vi "Handle Error.vi"(8 "error in (no error)":errorcluster, 11 "WebSocket Server in":refnum<class "WebSocket Server.lvclass">) -> (0 "error out":errorcluster, 2 "stop actor?":bool=TRUE, 3 "WebSocket Server out":refnum<class "WebSocket Server.lvclass">)   [LabVIEW 2021, in "WebSocket Actors.lvlib" / "WebSocket Server.lvclass"]
doc: "(<B>Filename</B>: Actor Framework.lvlib:Actor.lvclass:Handle Error.vi)\n\nDefines how the actor handles an error that occurred while processing a message. By default, this method does nothing except stop the actor."
uses:
  WebSocket Server.lvclass
  C:/Program Files/National Instruments/LabVIEW 2021/vi.lib/ActorFramework/Actor/Actor.lvclass
  <vilib>/ActorFramework/Actor/Actor.lvclass/Actor.ctl
  WebSocket Server.lvclass/WebSocket Server.ctl
  <vilib>/ActorFramework/Report Error Msg/Report Error Msg.lvclass/Report Error Msg.ctl
  <vilib>/ActorFramework/Message Enqueuer/Message Enqueuer.lvclass/Message Enqueuer.ctl
  Read Subscriber Enqueuer.vi
  <vilib>/ActorFramework/Message Enqueuer/Enqueue.vi
  <vilib>/ActorFramework/Message Enqueuer/Equals Not A Refnum.vi
  <vilib>/ActorFramework/Actor/Read Caller Enqueuer.vi
  <vilib>/ActorFramework/Report Error Msg/Report Error Msg.lvclass
  C:/Program Files/National Instruments/LabVIEW 2021/vi.lib/ActorFramework/Message/Message.lvclass
  <vilib>/Utility/LVClass/Get LV Class Name.vi
  <resource>/AFDebug/Generate Trace for Message.vi
  <vilib>/ActorFramework/Message Priority Queue/Priority Enqueue.vi
  <vilib>/ActorFramework/Message Enqueuer/Message Enqueuer.lvclass
  <userlib>/_OpenG.lib/error/error.llb/openg_error.lvlib
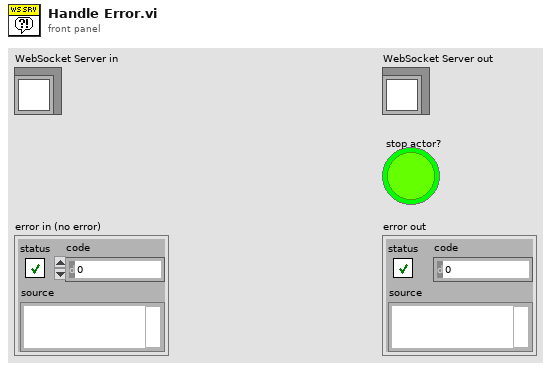
[diagram p1: front panel]
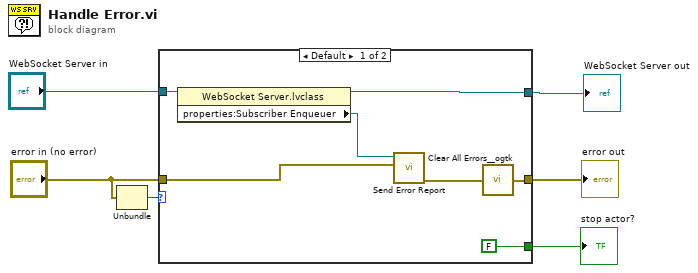
[diagram p0: block diagram]
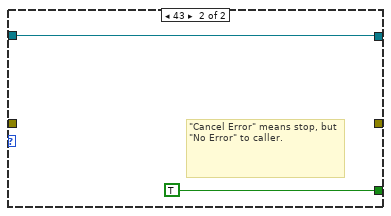
[diagram p2: hidden frame]
diagram:
  n1 = Unbundle("error in (no error)") -> ("code"=w6:i32)  [unwired: 2 out]
  n2 = case shown="Default" w6 {
    tunnel: [w8 _] -> w4
    tunnel: "error in (no error)" -> [w13 _]
    tunnel: [FALSE ("stop actor?") TRUE ("stop actor?")] -> w3
    tunnel: "WebSocket Server in" -> [w11 w14]
    tunnel: [w10 w14] -> w1
    frame Default {
      n3 = property class="WebSocket Server.lvclass"(reference=w11) -> (reference out=w10:refnum<class "WebSocket Server.lvclass">, "properties:Subscriber Enqueuer"=w9:refnum<class "Message Enqueuer.lvclass">)  [unwired: 1 in, 1 out]
      n4 = call <vilib>:"Send Error Report.vi"("Error From Sender"=w13, "Message Enqueuer"=w9) -> ("error out"=w7:errorcluster)  [unwired: 9 in]
      n5 = call <userlib>:"Clear All Errors__ogtk.vi"("Error In"=w7) -> ("Error Out"=w8:errorcluster)  [unwired: 3 in]
    }
    frame 43 {
      # "\"Cancel Error\" means stop, but \"No Error\" to caller."
    }
  }
  "WebSocket Server out" <- w1
  "error out" <- w4
  "stop actor?" <- w3
